vi "Thermometer.vi"() -> (0 "Temperature (deg F)":dbl(slide) scale=0.0..100.0)   [LabVIEW 2020]
panel:
  out "Reading (degC)":dbl
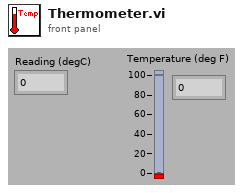
[diagram p1: front panel]
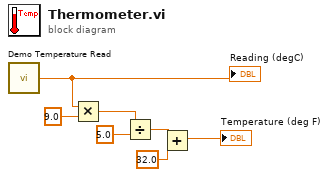
[diagram p0: block diagram]
diagram:
  n1 = call "Demo Temperature Read.vi"() -> ("Measured Temperature (degC)"=w7:dbl)  [unwired: 2 in]
  "Reading (degC)" <- w7
  n2 = Multiply(x=w7, y=9.0) -> (x*y=w5:dbl)
  n3 = Divide(x=w5, y=5.0) -> (x/y=w3:dbl)
  n4 = Add(x=w3, y=32.0) -> (x+y=→"Temperature (deg F)":dbl)
